vi "Open Account.vi"() -> (0 "sortie d'erreur":errorcluster, 3 "Infos sur le compte":T1)   [LabVIEW 2009]
uses:
  Account Info.ctl
  Stop.vi
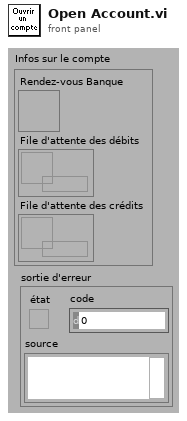
[diagram p1: front panel]
types:
  T1 = typedef "Account Info.ctl" = cluster{"Rendez-vous Banque":T2, "File d'attente des débits":refnum<queue>, "File d'attente des crédits":refnum<queue>}
  T2 = typedef "Rendezvous RefNum" = refnum<k1>
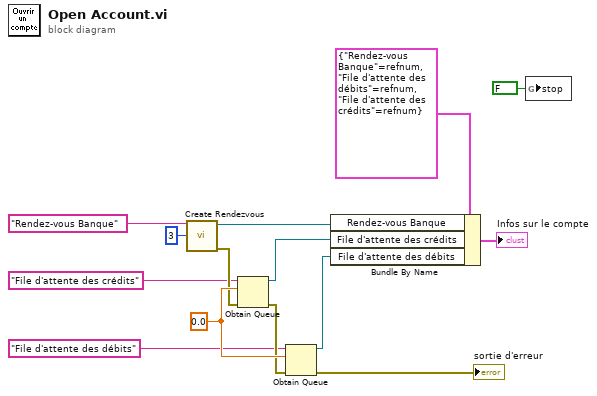
[diagram p0: block diagram]
diagram:
  w13 = 0.0
  n1 = call <vilib>:"Create Rendezvous.vi"("size (2)"=3, "name (unnamed)"="Rendez-vous Banque") -> ("error out"=w12:errorcluster, "rendezvous"=w14:T2)  [unwired: 1 in, 3 out]
  n2 = Obtain Queue ("Obtenir une file d'attente")(name (unnamed)="File d'attente des crédits", element data type=w13, error in (no error)=w12) -> (queue out=w10:refnum<queue>, error out=w11:errorcluster)  [unwired: 2 in, 1 out]
  n3 = Obtain Queue ("Obtenir une file d'attente")(name (unnamed)="File d'attente des débits", element data type=w13, error in (no error)=w11) -> (queue out=w9:refnum<queue>, error out=→"sortie d'erreur":errorcluster)  [unwired: 2 in, 1 out]
  n4 = Bundle By Name ("Assembler par nom")(cluster=T1 {"Rendez-vous Banque"=refnum, "File d'attente des débits"=refnum, "File d'attente des crédits"=refnum}, "Rendez-vous Banque"=w14, "File d'attente des crédits"=w10, "File d'attente des débits"=w9) -> (→"Infos sur le compte":T1)
  n5 = global write "Stop.vi" "stop"(FALSE ("stop")) -> ()
